vi "Handle Command.vi"(8 "error in (no error)":errorcluster, 9 "Data":variant, 10 "Command":string, 11 "Instrument in":refnum<class "Instrument.lvclass">) -> (0 "error out":errorcluster, 1 "Processed Data":variant, 2 "Command":string, 3 "Instrument out":refnum<class "Instrument.lvclass">)   [LabVIEW 2019, in "Instrument.lvclass"]
uses:
  Instrument.lvclass
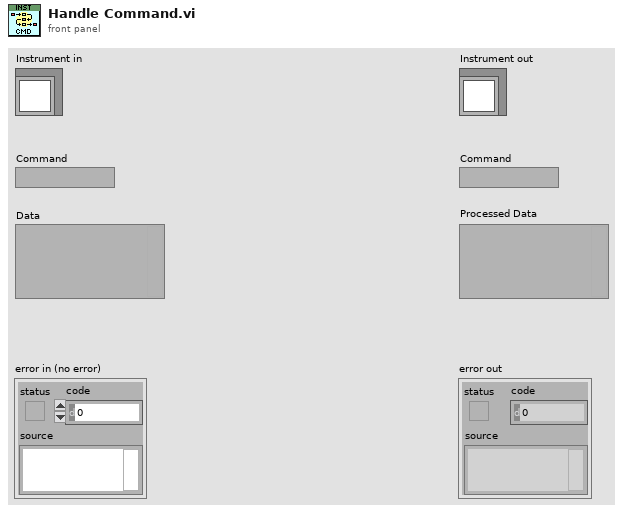
[diagram p1: front panel]
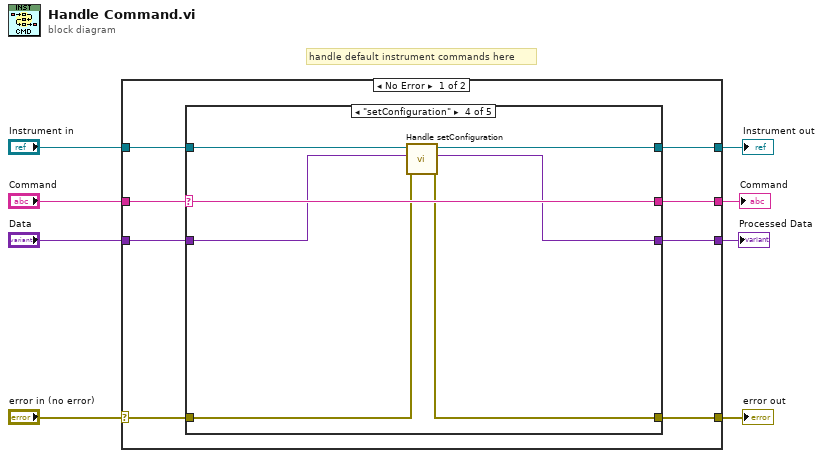
[diagram p0: block diagram]
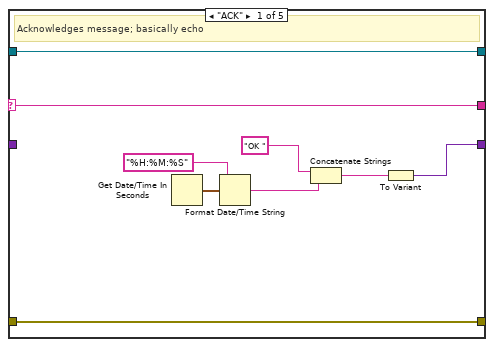
[diagram p2: hidden frame]
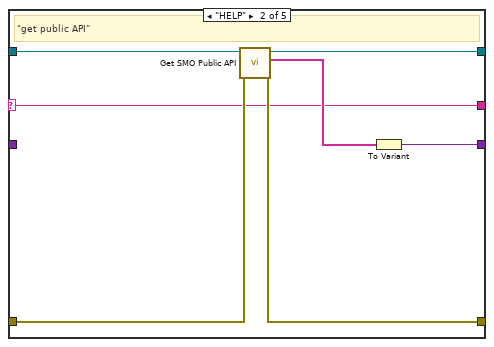
[diagram p3: hidden frame]
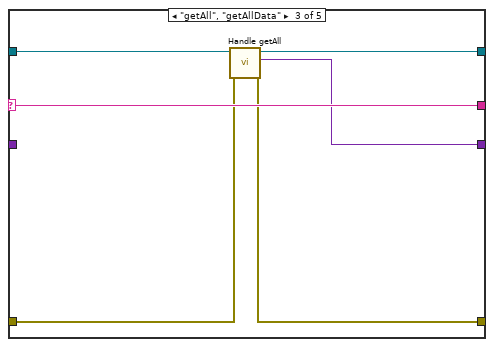
[diagram p4: hidden frame]
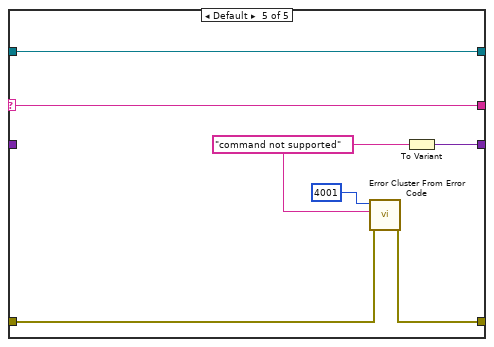
[diagram p5: hidden frame]
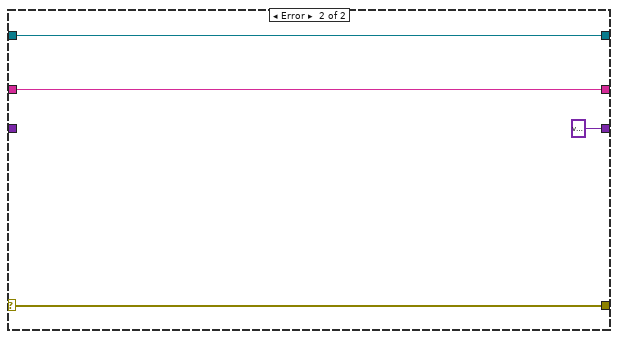
[diagram p6: hidden frame]
diagram:
  # "handle default instrument commands here"
  n1 = case shown="No Error" "error in (no error)" {
    selector: "error in (no error)" -> [w13 w55]
    tunnel: [w12 w55] -> w7
    tunnel: [w15 w54] -> w5
    tunnel: "Instrument in" -> [w16 w54]
    tunnel: "Command" -> [w10 w52]
    tunnel: [w14 variant ("error message (\"\")")] -> w4
    tunnel: "Data" -> [w9 _]
    tunnel: [w11 w52] -> w1
    frame No Error {
      n2 = case shown="\"setConfiguration\"" w10 {
        selector: w10 -> [w17 w26 w38 w44 w49]
        tunnel: w16 -> [w25 w32 w35 w41 w51]
        tunnel: [w25 w31 w34 w40 w51] -> w15
        tunnel: [w18 w30 w33 w39 w50] -> w14
        tunnel: w13 -> [w21 w28 w37 w43 w47]
        tunnel: [w21 w27 w36 w42 w46] -> w12
        tunnel: [w17 w26 w38 w44 w49] -> w11
        tunnel: w9 -> [_ _ _ w39 _]
        frame "ACK" {
          # "Acknowledges message; basically echo"
          n3 = Get Date/Time In Seconds() -> (seconds since 1Jan1904=w22:timestamp)
          n4 = Format Date/Time String(time format string (%c)="%H:%M:%S", seconds (now)=w22) -> (date/time string=w23:string)  [unwired: 1 in]
          n5 = Concatenate Strings("OK " ("data"), w23) -> (w20:string)
          n6 = To Variant(anything=w20) -> (Variant=w18:variant)
        }
        frame "HELP" {
          # "\"get public API\""
          n7 = call-dynamic "Get SMO Public API.vi"("error in (no error)"=w28, "Instrument in"=w32) -> ("error out"=w27:errorcluster, "Commands"=w29:string[], "Instrument out"=w31:refnum<class "Instrument.lvclass">)  [unwired: 7 in]
          n8 = To Variant(anything=w29) -> (Variant=w30:variant)
        }
        frame "getAll", "getAllData" {
          n9 = call-dynamic "Handle getAll.vi"("error in (no error)"=w37, "Instrument in"=w35) -> ("error out"=w36:errorcluster, "getAll"=w33:variant, "Instrument out"=w34:refnum<class "Instrument.lvclass">)  [unwired: 7 in]
        }
        frame "setConfiguration" {
          n10 = call-dynamic "Handle setConfiguration.vi"("error in (no error)"=w43, "setConfiguration"=w39, "Instrument in"=w41) -> ("error out"=w42:errorcluster, "Instrument out"=w40:refnum<class "Instrument.lvclass">)  [unwired: 7 in]
        }
        frame Default {
          w45 = "command not supported" ("error message (\"\")")
          n11 = call <vilib>:"Error Cluster From Error Code.vi"("error in (no error)"=w47, "error message (\"\")"=w45, "error code (0)"=4001) -> ("error out"=w46:errorcluster)  [unwired: 6 in]
          n12 = To Variant(anything=w45) -> (Variant=w50:variant)
        }
      }
    }
    frame Error {
    }
  }
  "error out" <- w7
  "Instrument out" <- w5
  "Processed Data" <- w4
  "Command" <- w1
